vi "main-all-channels.vi"() -> ()   [LabVIEW 2024]
uses:
  controls/thermocouple-input-cluster.ctl
  controls/analog-input-cluster.ctl
  controls/analog-output-cluster.ctl
  controls/digitial-input-cluster.ctl
  controls/digital-output-cluster.ctl
  controls/adam-module-select-tab.ctl
  controls/adam-5000-serial-settings.ctl
  controls/adam-5000-cmd-response.ctl
  controls/state-enum.ctl
  controls/adam-5000-all-chassis-data.ctl
  controls/adam-5000-all-module-datas.ctl
  controls/adam-5000-chassis-cmd-ack.ctl
  controls/adam-5000-chassis-module-types.ctl
  controls/adam-5000-DO-user-input.ctl
  controls/adam-5000-AO-user-input.ctl
  <vilib>/Instr/_visa.llb/VISA Configure Serial Port (Instr).vi
  <vilib>/Instr/_visa.llb/VISA Flush IO Buffer Mask.ctl
  controls/adam-5000-module-cmd-ack.ctl
panel:
  out "cmd-response:7":T1
  out "status-indicator:7":cluster{"Sampling":bool, "Ack":bool}
  in  "Slot 7: Module Type":T2(ring)=enum."empty"
  out "slot: 7":T3
  in  "7:Digital Outputs":T4
  out "7:Digital Inputs":T5
  in  "7:Analog Outputs":T6
  out "7:Analog Inputs":T7
  out "7:Thermocouple Inputs (degC)":T8
  out "cmd-response:6":T1
  out "status-indicator:6":cluster{"Sampling":bool, "Ack":bool}
  in  "Slot 6: Module Type":T2(ring)=enum."empty"
  out "slot: 6":T3
  in  "6:Digital Outputs":T4
  out "6:Digital Inputs":T5
  in  "6:Analog Outputs":T6
  out "6:Analog Inputs":T7
  out "6:Thermocouple Inputs (degC)":T8
  out "cmd-response:5":T1
  out "status-indicator:5":cluster{"Sampling":bool, "Ack":bool}
  in  "Slot 5: Module Type":T2(ring)=enum."Analog Output"
  out "slot: 5":T3
  in  "5:Digital Outputs":T4
  out "5:Digital Inputs":T5
  in  "5:Analog Outputs":T6
  out "5:Analog Inputs":T7
  out "5:Thermocouple Inputs (degC)":T8
  out "cmd-response:4":T1
  out "status-indicator:4":cluster{"Sampling":bool, "Ack":bool}
  in  "Slot 4: Module Type":T2(ring)=enum."Power Relay"
  out "slot: 4":T3
  in  "4:Digital Outputs":T4
  out "4:Digital Inputs":T5
  in  "4:Analog Outputs":T6
  out "4:Analog Inputs":T7
  out "4:Thermocouple Inputs (degC)":T8
  out "cmd-response:3":T1
  out "status-indicator:3":cluster{"Sampling":bool, "Ack":bool}
  in  "Slot 3: Module Type":T2(ring)=enum."Thermocouple"
  out "slot: 3":T3
  in  "3:Digital Outputs":T4
  out "3:Digital Inputs":T5
  in  "3:Analog Outputs":T6
  out "3:Analog Inputs":T7
  out "3:Thermocouple Inputs (degC)":T8
  out "cmd-response:2":T1
  out "status-indicator:2":cluster{"Sampling":bool, "Ack":bool}
  in  "Slot 2: Module Type":T2(ring)=enum."Analog Input"
  out "slot: 2":T3
  in  "2:Digital Outputs":T4
  out "2:Digital Inputs":T5
  in  "2:Analog Outputs":T6
  out "2:Analog Inputs":T7
  out "2:Thermocouple Inputs (degC)":T8
  out "cmd-response:1":T1
  out "status-indicator:1":cluster{"Sampling":bool, "Ack":bool}
  in  "Slot 1: Module Type":T2(ring)=enum."Thermocouple"
  out "slot: 1":T3
  in  "1:Digital Outputs":T4
  out "1:Digital Inputs":T5
  in  "1:Analog Outputs":T6
  out "1:Analog Inputs":T7
  out "1:Thermocouple Inputs (degC)":T8
  out "cmd-response:0":T1
  out "status-indicator:0":cluster{"Sampling":bool, "Ack":bool}
  in  "Slot 0: Module Type":T2(ring)=enum."Analog Input"
  out "slot: 0":T3
  in  "0:Digital Outputs":T4
  out "0:Digital Inputs":T5
  in  "0:Analog Outputs:":T6
  out "0:Analog Inputs":T7
  out "0:Thermocouple Inputs (degC)":T8
  out "Current Slot":i32
  in  "Chassis Settings":T9={"VISA resource name"="COM8", "baud rate (19200)"=19200, "Chassis ID"=1}
  in  "Debug Mode":bool
  out "Loop Time (mS)":u32
  out "Loop Counter":i32
  out "Write Success":bool
  out "error IO":errorcluster
  out "error":errorcluster
  in  "exit":bool
  # "ADAM 5000 Controller"
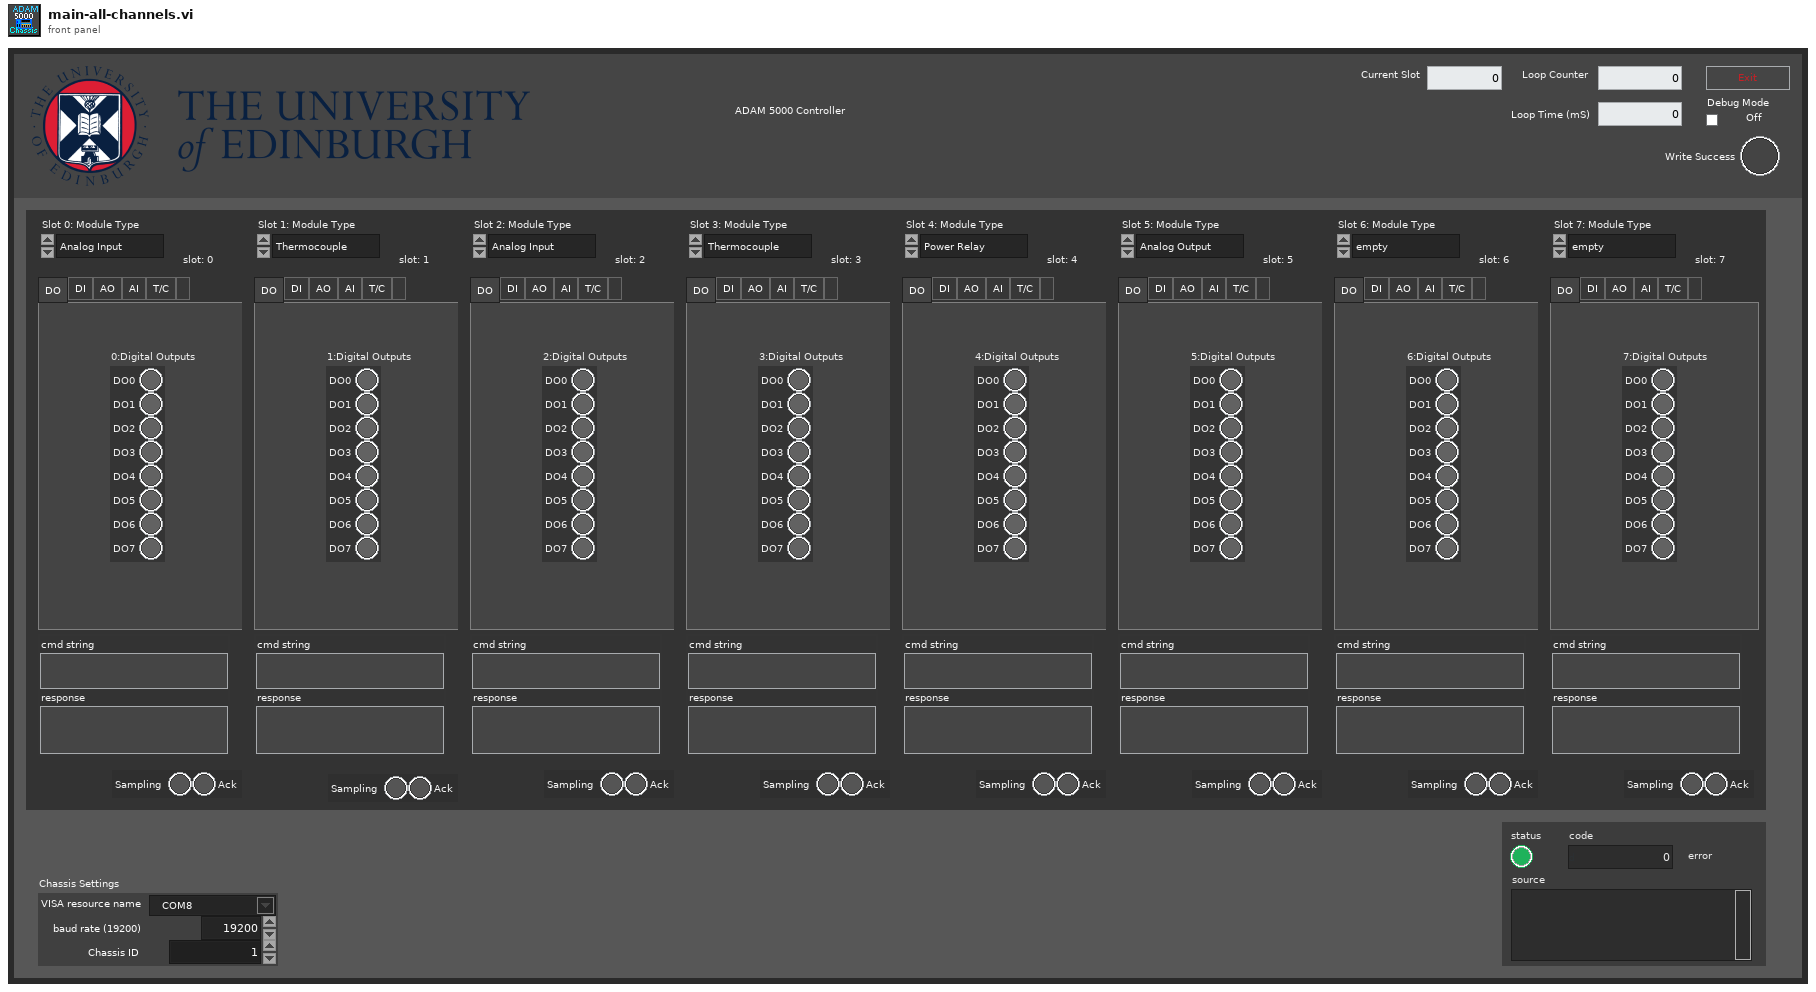
[diagram p1: front panel]
types:
  T1 = typedef "adam-5000-cmd-response.ctl" = cluster{"cmd string":string, "response":string}
  T2 = enum16{"Digital Output", "Digital Input", "Analog Output", "Analog Input", "Thermocouple", "Power Relay", "empty"}
  T3 = typedef "adam-module-select-tab.ctl" = enum32{"DO", "DI", "AO", "AI", "T/C", ""}
  T4 = typedef "digital-output-cluster.ctl" = cluster{"DO0":bool, "DO1":bool, "DO2":bool, "DO3":bool, "DO4":bool, "DO5":bool, "DO6":bool, "DO7":bool}
  T5 = typedef "digitial-input-cluster.ctl" = cluster{"DI0":bool, "DI1":bool, "DI2":bool, "DI3":bool, "DI4":bool, "DI5":bool, "DI6":bool, "DI7":bool}
  T6 = typedef "analog-output-cluster.ctl" = cluster{"AO0":dbl, "AO1":dbl, "AO2":dbl, "AO3":dbl}
  T7 = typedef "analog-input-cluster.ctl" = cluster{"AI0":dbl, "AI1":dbl, "AI2":dbl, "AI3":dbl, "AI4":dbl, "AI5":dbl, "AI6":dbl, "AI7":dbl}
  T8 = typedef "thermocouple-input-cluster.ctl" = cluster{"TC0":dbl, "TC1":dbl, "TC2":dbl, "TC3":dbl, "TC4":dbl, "TC5":dbl, "TC6":dbl}
  T9 = typedef "adam-5000-serial-settings.ctl" = cluster{"VISA resource name":refnum<visa-resource-name>, "baud rate (19200)":u32, "Chassis ID":u8}
  T10 = typedef "adam-5000-chassis-cmd-ack.ctl" = cluster{"cmd-response:0":T1, "cmd-response:1":T1, "cmd-response:2":T1, "cmd-response:3":T1, "cmd-response:4":T1, "cmd-response:5":T1, "cmd-response:6":T1, "cmd-response:7":T1}
  T11 = typedef "adam-5000-all-chassis-data.ctl" = cluster{"slot:0":T12, "slot:1":T12, "slot:2":T12, "slot:3":T12, "slot:4":T12, "slot:5":T12, "slot:6":T12, "slot:7":T12}
  T12 = typedef "adam-5000-all-module-datas.ctl" = cluster{"Digital Outputs":T4, "Digital Inputs":T5, "Analog Outputs":T6, "Analog Inputs":T7, "Thermocouple Inputs (degC)":T8}
  T13 = typedef "state-enum.ctl" = enum16{"init", "manual", "start", "run", "hold", "stop", ""}
  T14 = typedef "adam-5000-AO-user-input.ctl" = cluster{"0:Analog Outputs:":T6, "1:Analog Outputs":T6, "2:Analog Outputs":T6, "3:Analog Outputs":T6, "4:Analog Outputs":T6, "5:Analog Outputs":T6, "6:Analog Outputs":T6, "7:Analog Outputs":T6}
  T15 = typedef "adam-5000-DO-user-input.ctl" = cluster{"0:Digital Outputs":T4, "1:Digital Outputs":T4, "2:Digital Outputs":T4, "3:Digital Outputs":T4, "4:Digital Outputs":T4, "5:Digital Outputs":T4, "6:Digital Outputs":T4, "7:Digital Outputs":T4}
  T16 = typedef "adam-5000-chassis-module-types.ctl" = cluster{"Slot 0: Module Type":enum16{"Digital Output", "Digital Input", "Analog Output", "Analog Input", "Thermocouple", "Power Relay", "empty"}, "Slot 1: Module Type":enum16{"Digital Output", "Digital Input", "Analog Output", "Analog Input", "Thermocouple", "Power Relay", "empty"}, "Slot 2: Module Type":enum16{"Digital Output", "Digital Input", "Analog Output", "Analog Input", "Thermocouple", "Power Relay", "empty"}, "Slot 3: Module Type":enum16{"Digital Output", "Digital Input", "Analog Output", "Analog Input", "Thermocouple", "Power Relay", "empty"}, "Slot 4: Module Type":enum16{"Digital Output", "Digital Input", "Analog Output", "Analog Input", "Thermocouple", "Power Relay", "empty"}, "Slot 5: Module Type":enum16{"Digital Output", "Digital Input", "Analog Output", "Analog Input", "Thermocouple", "Power Relay", "empty"}, "Slot 6: Module Type":enum16{"Digital Output", "Digital Input", "Analog Output", "Analog Input", "Thermocouple", "Power Relay", "empty"}, "Slot 7: Module Type":enum16{"Digital Output", "Digital Input", "Analog Output", "Analog Input", "Thermocouple", "Power Relay", "empty"}}
  T17 = cluster{"status-indicator:0":refnum<vi>, "status-indicator:1":refnum<vi>, "status-indicator:2":refnum<vi>, "status-indicator:3":refnum<vi>, "status-indicator:4":refnum<vi>, "status-indicator:5":refnum<vi>, "status-indicator:6":refnum<vi>, "status-indicator:7":refnum<vi>}
  T18 = enum16{"Digital Output", "Digital Input", "Analog Output", "Analog Input", "Thermocouple", "Power Relay", "empty"}[]
  T19 = cluster{"[0]":T3, "[1]":T3, "[2]":T3, "[3]":T3, "[4]":T3, "[5]":T3, "[6]":T3, "[7]":T3, "[8]":T3}
  T20 = cluster{"[0]":T12, "[1]":T12, "[2]":T12, "[3]":T12, "[4]":T12, "[5]":T12, "[6]":T12, "[7]":T12, "[8]":T12}
  T21 = cluster{"[0]":T1, "[1]":T1, "[2]":T1, "[3]":T1, "[4]":T1, "[5]":T1, "[6]":T1, "[7]":T1, "[8]":T1}
  T22 = typedef "adam-5000-module-cmd-ack.ctl" = cluster{"cmd out":string, "acknowledge char":string}
  T23 = cluster{"[0]":T22, "[1]":T22, "[2]":T22, "[3]":T22, "[4]":T22, "[5]":T22, "[6]":T22, "[7]":T22, "[8]":T22}
  T24 = typedef "VISA Flush IO Buffer Mask.ctl" = u16
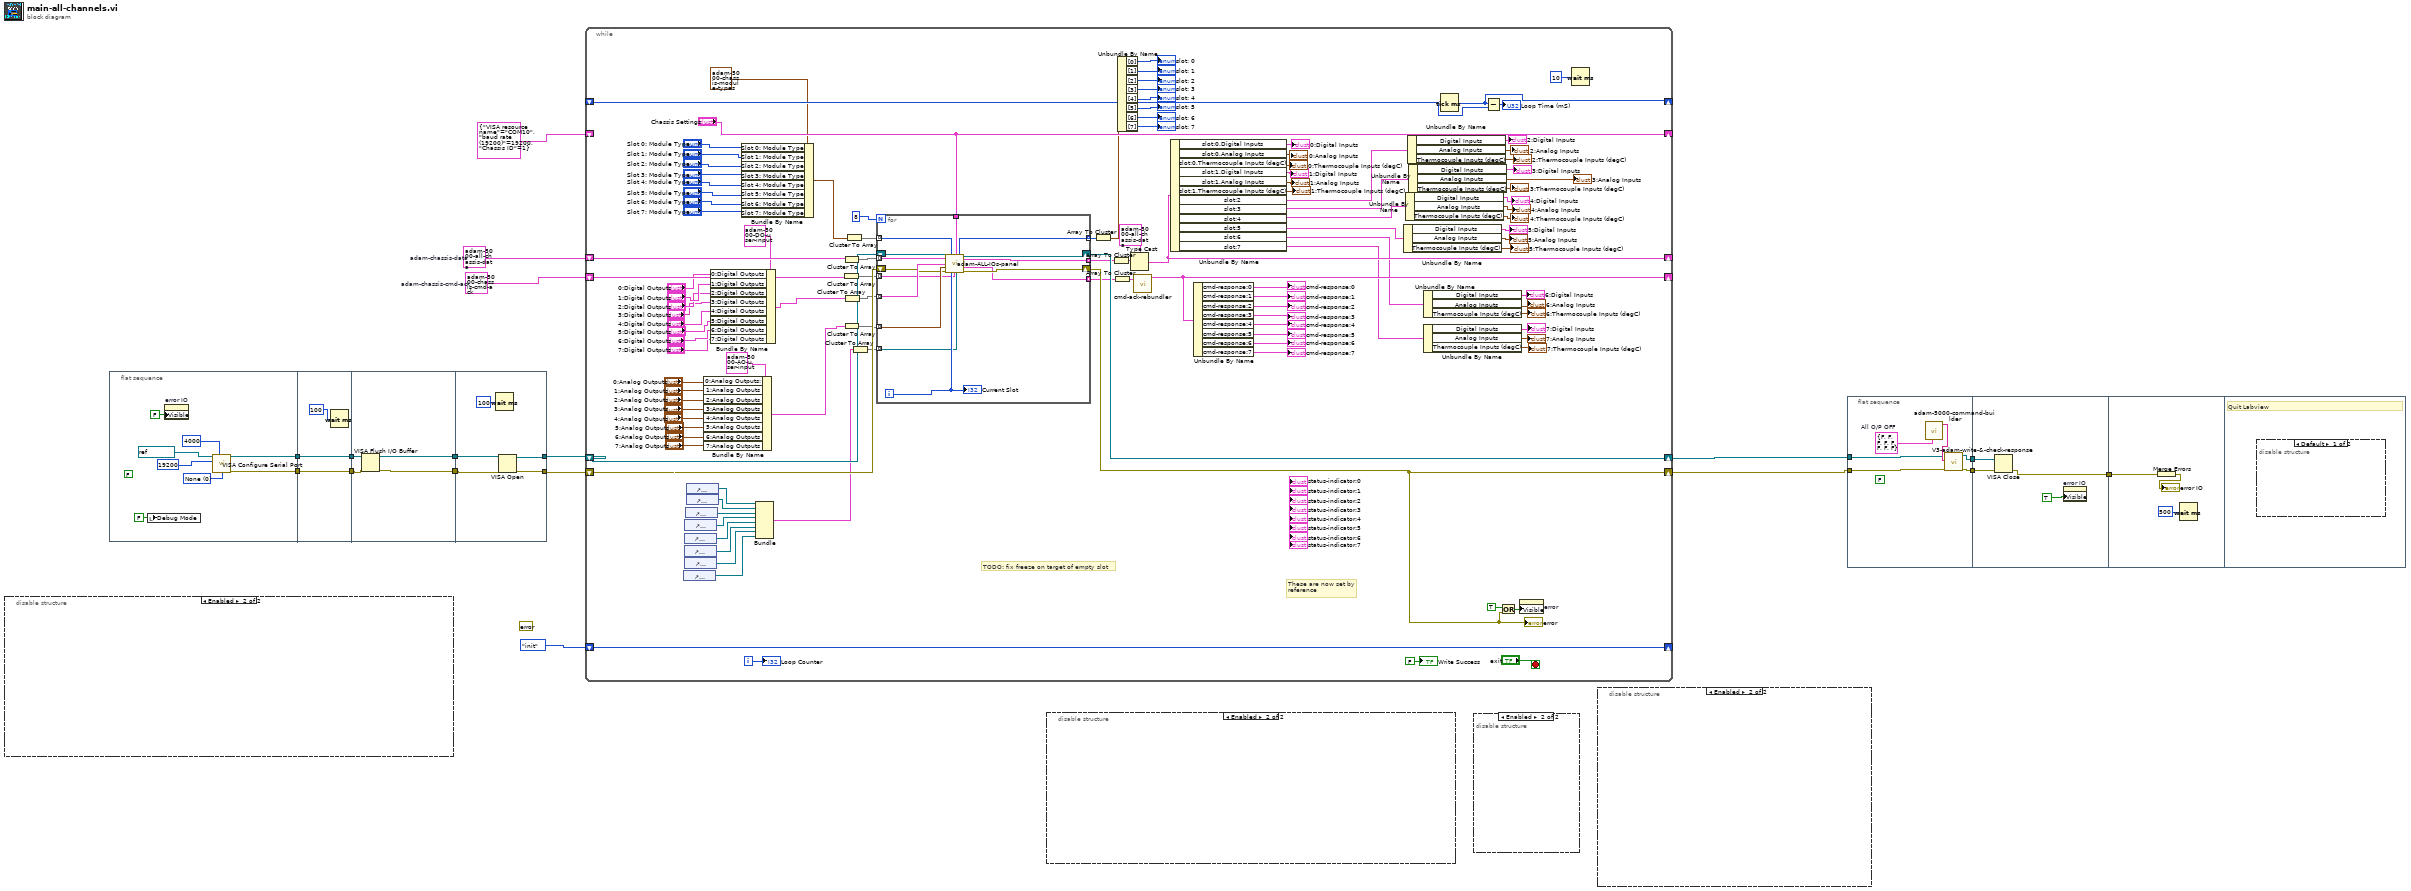
[diagram p0: block diagram]
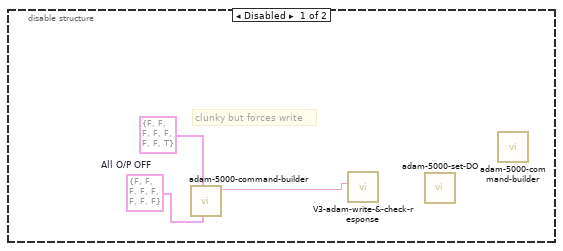
[diagram p2: hidden frame]
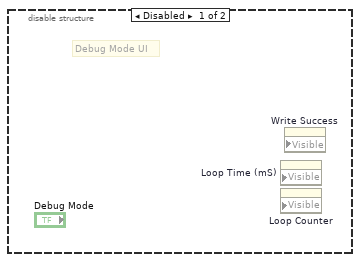
[diagram p3: hidden frame]
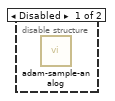
[diagram p4: hidden frame]
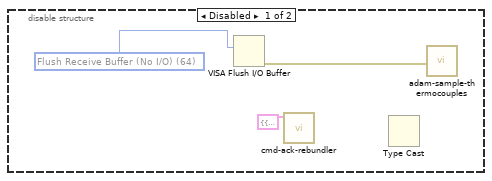
[diagram p5: hidden frame]
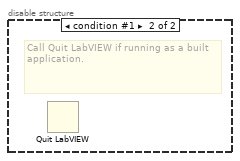
[diagram p6: hidden frame]
diagram:
  w1 = T10 {"cmd-response:0"={"cmd string"="", "response"=""}, "cmd-response:1"={"cmd string"="", "response"=""}, "cmd-response:2"={"cmd string"="", "response"=""}, "cmd-response:3"={"cmd string"="", "response"=""}, "cmd-response:4"={"cmd string"="", "response"=""}, "cmd-response:5"={"cmd string"="", "response"=""}, "cmd-response:6"={"cmd string"="", "response"=""}, "cmd-response:7"={"cmd string"="", "response"=""}}  # adam-chassis-cmd-ack
  w2 = T11 {"slot:0"={"Digital Outputs"={"DO0"=FALSE, "DO1"=FALSE, "DO2"=FALSE, "DO3"=FALSE, "DO4"=FALSE, "DO5"=FALSE, "DO6"=FALSE, "DO7"=FALSE}, "Digital Inputs"={"DI0"=FALSE, "DI1"=FALSE, "DI2"=FALSE, "DI3"=FALSE, "DI4"=FALSE, "DI5"=FALSE, "DI6"=FALSE, "DI7"=FALSE}, "Analog Outputs"={"AO0"=0.0, "AO1"=0.0, "AO2"=0.0, "AO3"=0.0}, "Analog Inputs"={"AI0"=0.0, "AI1"=0.0, "AI2"=0.0, "AI3"=0.0, "AI4"=0.0, "AI5"=0.0, "AI6"=0.0, "AI7"=0.0}, "Thermocouple Inputs (degC)"={"TC0"=0.0, "TC1"=0.0, "TC2"=0.0, "TC3"=0.0, "TC4"=0.0, "TC5"=0.0, "TC6"=0.0}}, "slot:1"={"Digital Outputs"={"DO0"=FALSE, "DO1"=FALSE, "DO2"=FALSE, "DO3"=FALSE, "DO4"=FALSE, "DO5"=FALSE, "DO6"=FALSE, "DO7"=FALSE}, "Digital Inputs"={"DI0"=FALSE, "DI1"=FALSE, "DI2"=FALSE, "DI3"=FALSE, "DI4"=FALSE, "DI5"=FALSE, "DI6"=FALSE, "DI7"=FALSE}, "Analog Outputs"={"AO0"=0.0, "AO1"=0.0, "AO2"=0.0, "AO3"=0.0}, "Analog Inputs"={"AI0"=0.0, "AI1"=0.0, "AI2"=0.0, "AI3"=0.0, "AI4"=0.0, "AI5"=0.0, "AI6"=0.0, "AI7"=0.0}, "Thermocouple Inputs (degC)"={"TC0"=0.0, "TC1"=0.0, "TC2"=0.0, "TC3"=0.0, "TC4"=0.0, "TC5"=0.0, "TC6"=0.0}}, "slot:2"={"Digital Outputs"={"DO0"=FALSE, "DO1"=FALSE, "DO2"=FALSE, "DO3"=FALSE, "DO4"=FALSE, "DO5"=FALSE, "DO6"=FALSE, "DO7"=FALSE}, "Digital Inputs"={"DI0"=FALSE, "DI1"=FALSE, "DI2"=FALSE, "DI3"=FALSE, "DI4"=FALSE, "DI5"=FALSE, "DI6"=FALSE, "DI7"=FALSE}, "Analog Outputs"={"AO0"=0.0, "AO1"=0.0, "AO2"=0.0, "AO3"=0.0}, "Analog Inputs"={"AI0"=0.0, "AI1"=0.0, "AI2"=0.0, "AI3"=0.0, "AI4"=0.0, "AI5"=0.0, "AI6"=0.0, "AI7"=0.0}, "Thermocouple Inputs (degC)"={"TC0"=0.0, "TC1"=0.0, "TC2"=0.0, "TC3"=0.0, "TC4"=0.0, "TC5"=0.0, "TC6"=0.0}}, "slot:3"={"Digital Outputs"={"DO0"=FALSE, "DO1"=FALSE, "DO2"=FALSE, "DO3"=FALSE, "DO4"=FALSE, "DO5"=FALSE, "DO6"=FALSE, "DO7"=FALSE}, "Digital Inputs"={"DI0"=FALSE, "DI1"=FALSE, "DI2"=FALSE, "DI3"=FALSE, "DI4"=FALSE, "DI5"=FALSE, "DI6"=FALSE, "DI7"=FALSE}, "Analog Outputs"={"AO0"=0.0, "AO1"=0.0, "AO2"=0.0, "AO3"=0.0}, "Analog Inputs"={"AI0"=0.0, "AI1"=0.0, "AI2"=0.0, "AI3"=0.0, "AI4"=0.0, "AI5"=0.0, "AI6"=0.0, "AI7"=0.0}, "Thermocouple Inputs (degC)"={"TC0"=0.0, "TC1"=0.0, "TC2"=0.0, "TC3"=0.0, "TC4"=0.0, "TC5"=0.0, "TC6"=0.0}}, "slot:4"={"Digital Outputs"={"DO0"=FALSE, "DO1"=FALSE, "DO2"=FALSE, "DO3"=FALSE, "DO4"=FALSE, "DO5"=FALSE, "DO6"=FALSE, "DO7"=FALSE}, "Digital Inputs"={"DI0"=FALSE, "DI1"=FALSE, "DI2"=FALSE, "DI3"=FALSE, "DI4"=FALSE, "DI5"=FALSE, "DI6"=FALSE, "DI7"=FALSE}, "Analog Outputs"={"AO0"=0.0, "AO1"=0.0, "AO2"=0.0, "AO3"=0.0}, "Analog Inputs"={"AI0"=0.0, "AI1"=0.0, "AI2"=0.0, "AI3"=0.0, "AI4"=0.0, "AI5"=0.0, "AI6"=0.0, "AI7"=0.0}, "Thermocouple Inputs (degC)"={"TC0"=0.0, "TC1"=0.0, "TC2"=0.0, "TC3"=0.0, "TC4"=0.0, "TC5"=0.0, "TC6"=0.0}}, "slot:5"={"Digital Outputs"={"DO0"=FALSE, "DO1"=FALSE, "DO2"=FALSE, "DO3"=FALSE, "DO4"=FALSE, "DO5"=FALSE, "DO6"=FALSE, "DO7"=FALSE}, "Digital Inputs"={"DI0"=FALSE, "DI1"=FALSE, "DI2"=FALSE, "DI3"=FALSE, "DI4"=FALSE, "DI5"=FALSE, "DI6"=FALSE, "DI7"=FALSE}, "Analog Outputs"={"AO0"=0.0, "AO1"=0.0, "AO2"=0.0, "AO3"=0.0}, "Analog Inputs"={"AI0"=0.0, "AI1"=0.0, "AI2"=0.0, "AI3"=0.0, "AI4"=0.0, "AI5"=0.0, "AI6"=0.0, "AI7"=0.0}, "Thermocouple Inputs (degC)"={"TC0"=0.0, "TC1"=0.0, "TC2"=0.0, "TC3"=0.0, "TC4"=0.0, "TC5"=0.0, "TC6"=0.0}}, "slot:6"={"Digital Outputs"={"DO0"=FALSE, "DO1"=FALSE, "DO2"=FALSE, "DO3"=FALSE, "DO4"=FALSE, "DO5"=FALSE, "DO6"=FALSE, "DO7"=FALSE}, "Digital Inputs"={"DI0"=FALSE, "DI1"=FALSE, "DI2"=FALSE, "DI3"=FALSE, "DI4"=FALSE, "DI5"=FALSE, "DI6"=FALSE, "DI7"=FALSE}, "Analog Outputs"={"AO0"=0.0, "AO1"=0.0, "AO2"=0.0, "AO3"=0.0}, "Analog Inputs"={"AI0"=0.0, "AI1"=0.0, "AI2"=0.0, "AI3"=0.0, "AI4"=0.0, "AI5"=0.0, "AI6"=0.0, "AI7"=0.0}, "Thermocouple Inputs (degC)"={"TC0"=0.0, "TC1"=0.0, "TC2"=0.0, "TC3"=0.0, "TC4"=0.0, "TC5"=0.0, "TC6"=0.0}}, "slot:7"={"Digital Outputs"={"DO0"=FALSE, "DO1"=FALSE, "DO2"=FALSE, "DO3"=FALSE, "DO4"=FALSE, "DO5"=FALSE, "DO6"=FALSE, "DO7"=FALSE}, "Digital Inputs"={"DI0"=FALSE, "DI1"=FALSE, "DI2"=FALSE, "DI3"=FALSE, "DI4"=FALSE, "DI5"=FALSE, "DI6"=FALSE, "DI7"=FALSE}, "Analog Outputs"={"AO0"=0.0, "AO1"=0.0, "AO2"=0.0, "AO3"=0.0}, "Analog Inputs"={"AI0"=0.0, "AI1"=0.0, "AI2"=0.0, "AI3"=0.0, "AI4"=0.0, "AI5"=0.0, "AI6"=0.0, "AI7"=0.0}, "Thermocouple Inputs (degC)"={"TC0"=0.0, "TC1"=0.0, "TC2"=0.0, "TC3"=0.0, "TC4"=0.0, "TC5"=0.0, "TC6"=0.0}}}  # adam-chassis-data
  (unwired) errorcluster {"status"=FALSE, "code"=0, "source"=""} ("error")
  n1 = disable-structure shown="Enabled" {
    frame Disabled {
      w20 = T4 {"DO0"=FALSE, "DO1"=FALSE, "DO2"=FALSE, "DO3"=FALSE, "DO4"=FALSE, "DO5"=FALSE, "DO6"=FALSE, "DO7"=FALSE}  # All O/P OFF
      # "clunky but forces write"
      n2 = call "adam-5000-command-builder.vi"("Output Control"=w20, "Current Output State"=T4 {"DO0"=FALSE, "DO1"=FALSE, "DO2"=FALSE, "DO3"=FALSE, "DO4"=FALSE, "DO5"=FALSE, "DO6"=FALSE, "DO7"=TRUE}) -> ("Command Out"=w19:string)  [unwired: 7 in, 2 out]
      n3 = call "V3-adam-write-&-check-response.vi"("write buffer"=w19) -> ("VISA resource name"=w18:refnum<visa-resource-name>)  [unwired: 5 in, 5 out]
      n4 = call "adam-5000-set-DO.vi"() -> ()  [unwired: 6 in, 6 out]
      n5 = call "adam-5000-command-builder.vi"() -> ()  [unwired: 9 in, 3 out]
    }
    frame Enabled {
    }
  }
  n6 = flat-sequence {
    tunnel: [w28] -> w11
    tunnel: [w27] -> w10
    tunnel: w11 -> [w32]
    tunnel: [w32] -> w9
    tunnel: w10 -> [w31]
    tunnel: [w31] -> w8
    tunnel: w9 -> [w36]
    tunnel: [w34] -> w7
    tunnel: w8 -> [w35]
    tunnel: [w33] -> w6
    tunnel: w7 -> [w40]
    tunnel: w6 -> [w39]
    tunnel: [w38] -> w5
    tunnel: [w37] -> w4
    frame #0 {
      w25 = u16 0 items=["None", "XON/XOFF", "RTS/CTS", "XON/XOFF & RTS/CTS", "DTR/DSR", "XON/XOFF & DTR/DSR"] ("flow control (0:none)")
      (unwired) FALSE ("V1")
      n7 = local write "Debug Mode"(FALSE ("Debug Mode")) -> ()
      n8 = property on="error IO" class="Clust (strict)"("Visible"=FALSE) -> ()  [unwired: 2 in, 2 out]
      n9 = call-poly "VISA Configure Serial Port"("VISA resource name"=refnum<visa-resource-name> "COM8", "timeout (10sec)"=u32 4000, "baud rate (9600)"=u32 19200, "flow control (0:none)"=w25) -> ("VISA resource name out"=w28:refnum<visa-resource-name>, "error out"=w27:errorcluster)  [unwired: 10 in]
    }
    frame #1 {
      n10 = Wait (ms)(milliseconds to wait=u32 100) -> ()  [unwired: 1 out]
    }
    frame #2 {
      n11 = VISA Flush I/O Buffer(VISA resource name=w36, error in (no error)=w35) -> (VISA resource name out=w34:refnum<visa-resource-name>, error out=w33:errorcluster)  [unwired: 1 in]
    }
    frame #3 {
      n12 = Wait (ms)(milliseconds to wait=u32 100) -> ()  [unwired: 1 out]
      n13 = VISA Open(error in (no error)=w39, VISA resource name=w40) -> (VISA resource name=w38:refnum<visa-resource-name>, error out=w37:errorcluster)  [unwired: 3 in]
    }
  }
  n14 = while {
    shift-right: [w151] -> _
    shift-left: state-enum."init" ("state-enum") -> [w151]
    shift-right: [w127] -> w16
    shift-left: w4 -> [w139]
    shift-right: [w154] -> _
    shift-left: _ -> [w156]
    shift-right: ["Chassis Settings"] -> _
    shift-left: T9 {"VISA resource name"="COM10", "baud rate (19200)"=19200, "Chassis ID"=1} ("Chassis Settings") -> [_]
    shift-right: [w138] -> w3
    shift-left: w5 -> [w140]
    shift-right: [w128] -> _
    shift-left: w2 -> [w137]
    shift-right: [w112] -> _
    shift-left: w1 -> [w135]
    i -> [w157]
    stop <- "exit" stop-if-true
    # "TODO: fix freeze on target of empty slot"
    # "These are now set by\nreference"
    n15 = control-ref of="status-indicator:7"() -> (w72:refnum<vi>)
    n16 = control-ref of="status-indicator:4"() -> (w75:refnum<vi>)
    n17 = control-ref of="status-indicator:5"() -> (w74:refnum<vi>)
    n18 = control-ref of="status-indicator:3"() -> (w76:refnum<vi>)
    n19 = control-ref of="status-indicator:6"() -> (w73:refnum<vi>)
    n20 = control-ref of="status-indicator:2"() -> (w106:refnum<vi>)
    n21 = control-ref of="status-indicator:0"() -> (w124:refnum<vi>)
    n22 = control-ref of="status-indicator:1"() -> (w123:refnum<vi>)
    n23 = Bundle By Name(cluster=T14 {"0:Analog Outputs:"={"AO0"=0.0, "AO1"=0.0, "AO2"=0.0, "AO3"=0.0}, "1:Analog Outputs"={"AO0"=0.0, "AO1"=0.0, "AO2"=0.0, "AO3"=0.0}, "2:Analog Outputs"={"AO0"=0.0, "AO1"=0.0, "AO2"=0.0, "AO3"=0.0}, "3:Analog Outputs"={"AO0"=0.0, "AO1"=0.0, "AO2"=0.0, "AO3"=0.0}, "4:Analog Outputs"={"AO0"=0.0, "AO1"=0.0, "AO2"=0.0, "AO3"=0.0}, "5:Analog Outputs"={"AO0"=0.0, "AO1"=0.0, "AO2"=0.0, "AO3"=0.0}, "6:Analog Outputs"={"AO0"=0.0, "AO1"=0.0, "AO2"=0.0, "AO3"=0.0}, "7:Analog Outputs"={"AO0"=0.0, "AO1"=0.0, "AO2"=0.0, "AO3"=0.0}}, "0:Analog Outputs:"="0:Analog Outputs:", "1:Analog Outputs"="1:Analog Outputs", "2:Analog Outputs"="2:Analog Outputs", "3:Analog Outputs"="3:Analog Outputs", "4:Analog Outputs"="4:Analog Outputs", "5:Analog Outputs"="5:Analog Outputs", "6:Analog Outputs"="6:Analog Outputs", "7:Analog Outputs"="7:Analog Outputs") -> (w50:T14)
    n24 = Bundle By Name(cluster=T15 {"0:Digital Outputs"={"DO0"=FALSE, "DO1"=FALSE, "DO2"=FALSE, "DO3"=FALSE, "DO4"=FALSE, "DO5"=FALSE, "DO6"=FALSE, "DO7"=FALSE}, "1:Digital Outputs"={"DO0"=FALSE, "DO1"=FALSE, "DO2"=FALSE, "DO3"=FALSE, "DO4"=FALSE, "DO5"=FALSE, "DO6"=FALSE, "DO7"=FALSE}, "2:Digital Outputs"={"DO0"=FALSE, "DO1"=FALSE, "DO2"=FALSE, "DO3"=FALSE, "DO4"=FALSE, "DO5"=FALSE, "DO6"=FALSE, "DO7"=FALSE}, "3:Digital Outputs"={"DO0"=FALSE, "DO1"=FALSE, "DO2"=FALSE, "DO3"=FALSE, "DO4"=FALSE, "DO5"=FALSE, "DO6"=FALSE, "DO7"=FALSE}, "4:Digital Outputs"={"DO0"=FALSE, "DO1"=FALSE, "DO2"=FALSE, "DO3"=FALSE, "DO4"=FALSE, "DO5"=FALSE, "DO6"=FALSE, "DO7"=FALSE}, "5:Digital Outputs"={"DO0"=FALSE, "DO1"=FALSE, "DO2"=FALSE, "DO3"=FALSE, "DO4"=FALSE, "DO5"=FALSE, "DO6"=FALSE, "DO7"=FALSE}, "6:Digital Outputs"={"DO0"=FALSE, "DO1"=FALSE, "DO2"=FALSE, "DO3"=FALSE, "DO4"=FALSE, "DO5"=FALSE, "DO6"=FALSE, "DO7"=FALSE}, "7:Digital Outputs"={"DO0"=FALSE, "DO1"=FALSE, "DO2"=FALSE, "DO3"=FALSE, "DO4"=FALSE, "DO5"=FALSE, "DO6"=FALSE, "DO7"=FALSE}}, "0:Digital Outputs"="0:Digital Outputs", "1:Digital Outputs"="1:Digital Outputs", "2:Digital Outputs"="2:Digital Outputs", "3:Digital Outputs"="3:Digital Outputs", "4:Digital Outputs"="4:Digital Outputs", "5:Digital Outputs"="5:Digital Outputs", "6:Digital Outputs"="6:Digital Outputs", "7:Digital Outputs"="7:Digital Outputs") -> (w60:T15)
    n25 = Bundle By Name(cluster=T16 {"Slot 0: Module Type"=enum."Digital Output", "Slot 1: Module Type"=enum."Digital Output", "Slot 2: Module Type"=enum."Digital Output", "Slot 3: Module Type"=enum."Digital Output", "Slot 4: Module Type"=enum."Digital Output", "Slot 5: Module Type"=enum."Digital Output", "Slot 6: Module Type"=enum."Digital Output", "Slot 7: Module Type"=enum."Digital Output"}, "Slot 0: Module Type"="Slot 0: Module Type", "Slot 1: Module Type"="Slot 1: Module Type", "Slot 2: Module Type"="Slot 2: Module Type", "Slot 3: Module Type"="Slot 3: Module Type", "Slot 4: Module Type"="Slot 4: Module Type", "Slot 5: Module Type"="Slot 5: Module Type", "Slot 6: Module Type"="Slot 6: Module Type", "Slot 7: Module Type"="Slot 7: Module Type") -> (w62:T16)
    n26 = Bundle("status-indicator:0"=w124, "status-indicator:1"=w123, "status-indicator:2"=w106, "status-indicator:3"=w76, "status-indicator:4"=w75, "status-indicator:5"=w74, "status-indicator:6"=w73, "status-indicator:7"=w72) -> (w122:T17)  [unwired: 1 in]
    n27 = Cluster To Array(cluster=w135) -> (array=w134:T1[])
    n28 = Cluster To Array(cluster=w137) -> (array=w136:T12[])
    n29 = Cluster To Array(cluster=w50) -> (array=w132:T6[])
    n30 = Cluster To Array(cluster=w60) -> (array=w133:T4[])
    n31 = Cluster To Array(cluster=w62) -> (array=w126:T18)
    n32 = Cluster To Array(cluster=w122) -> (array=w121:refnum<vi>[])
    n33 = for {
      N: 8 -> [_]
      shift-right: [w165] -> w127
      shift-left: w139 -> [w166]
      shift-right: [w171] -> w138
      shift-left: w140 -> [w170]
      tunnel: w136 -> [w169] mode=indexing
      tunnel: w134 -> [w161] mode=indexing
      tunnel: w133 -> [w168] mode=indexing
      tunnel: w132 -> [w167] mode=indexing
      tunnel: "Chassis Settings" -> [w173]
      tunnel: w126 -> [w174] mode=indexing
      tunnel: w121 -> [w160] mode=indexing
      tunnel: [w172] -> w120 mode=indexing
      tunnel: [w164] -> w119 mode=indexing
      tunnel: [w163] -> w118 mode=indexing
      i -> [w162]
      n34 = call "adam-ALL-IOs-panel.vi"("VISA Refnum in"=w170, "ADAM-5000-data-current"=w169, "Digital Outputs"=w168, "Analog Outputs"=w167, "error in (no error)"=w166, "Module Type"=w174, "chassis-slot"=w162, "cmd-response in"=w161, "Chassis Settings"=w173, "reference"=w160) -> ("slot: x"=w172:T3, "VISA Refnum out"=w171:refnum<visa-resource-name>, "ADAM-5000-data-new"=w164:T12, "cmd-response out"=w163:T1, "error out"=w165:errorcluster)  [unwired: 5 in]
      "Current Slot" <- w162
    }
    "error" <- w127
    n35 = Array To Cluster(array=w120) -> (cluster=w125:T19)
    n36 = Array To Cluster(array=w119) -> (cluster=w130:T20)
    n37 = Array To Cluster(array=w118) -> (cluster=w111:T21)
    n38 = Unbundle By Name(w125) -> ("[0]"=→"slot: 0":T3, "[1]"=→"slot: 1":T3, "[2]"=→"slot: 2":T3, "[3]"=→"slot: 3":T3, "[4]"=→"slot: 4":T3, "[5]"=→"slot: 5":T3, "[6]"=→"slot: 6":T3, "[7]"=→"slot: 7":T3)
    n39 = Type Cast(type=T11 {"slot:0"={"Digital Outputs"={"DO0"=FALSE, "DO1"=FALSE, "DO2"=FALSE, "DO3"=FALSE, "DO4"=FALSE, "DO5"=FALSE, "DO6"=FALSE, "DO7"=FALSE}, "Digital Inputs"={"DI0"=FALSE, "DI1"=FALSE, "DI2"=FALSE, "DI3"=FALSE, "DI4"=FALSE, "DI5"=FALSE, "DI6"=FALSE, "DI7"=FALSE}, "Analog Outputs"={"AO0"=0.0, "AO1"=0.0, "AO2"=0.0, "AO3"=0.0}, "Analog Inputs"={"AI0"=0.0, "AI1"=0.0, "AI2"=0.0, "AI3"=0.0, "AI4"=0.0, "AI5"=0.0, "AI6"=0.0, "AI7"=0.0}, "Thermocouple Inputs (degC)"={"TC0"=0.0, "TC1"=0.0, "TC2"=0.0, "TC3"=0.0, "TC4"=0.0, "TC5"=0.0, "TC6"=0.0}}, "slot:1"={"Digital Outputs"={"DO0"=FALSE, "DO1"=FALSE, "DO2"=FALSE, "DO3"=FALSE, "DO4"=FALSE, "DO5"=FALSE, "DO6"=FALSE, "DO7"=FALSE}, "Digital Inputs"={"DI0"=FALSE, "DI1"=FALSE, "DI2"=FALSE, "DI3"=FALSE, "DI4"=FALSE, "DI5"=FALSE, "DI6"=FALSE, "DI7"=FALSE}, "Analog Outputs"={"AO0"=0.0, "AO1"=0.0, "AO2"=0.0, "AO3"=0.0}, "Analog Inputs"={"AI0"=0.0, "AI1"=0.0, "AI2"=0.0, "AI3"=0.0, "AI4"=0.0, "AI5"=0.0, "AI6"=0.0, "AI7"=0.0}, "Thermocouple Inputs (degC)"={"TC0"=0.0, "TC1"=0.0, "TC2"=0.0, "TC3"=0.0, "TC4"=0.0, "TC5"=0.0, "TC6"=0.0}}, "slot:2"={"Digital Outputs"={"DO0"=FALSE, "DO1"=FALSE, "DO2"=FALSE, "DO3"=FALSE, "DO4"=FALSE, "DO5"=FALSE, "DO6"=FALSE, "DO7"=FALSE}, "Digital Inputs"={"DI0"=FALSE, "DI1"=FALSE, "DI2"=FALSE, "DI3"=FALSE, "DI4"=FALSE, "DI5"=FALSE, "DI6"=FALSE, "DI7"=FALSE}, "Analog Outputs"={"AO0"=0.0, "AO1"=0.0, "AO2"=0.0, "AO3"=0.0}, "Analog Inputs"={"AI0"=0.0, "AI1"=0.0, "AI2"=0.0, "AI3"=0.0, "AI4"=0.0, "AI5"=0.0, "AI6"=0.0, "AI7"=0.0}, "Thermocouple Inputs (degC)"={"TC0"=0.0, "TC1"=0.0, "TC2"=0.0, "TC3"=0.0, "TC4"=0.0, "TC5"=0.0, "TC6"=0.0}}, "slot:3"={"Digital Outputs"={"DO0"=FALSE, "DO1"=FALSE, "DO2"=FALSE, "DO3"=FALSE, "DO4"=FALSE, "DO5"=FALSE, "DO6"=FALSE, "DO7"=FALSE}, "Digital Inputs"={"DI0"=FALSE, "DI1"=FALSE, "DI2"=FALSE, "DI3"=FALSE, "DI4"=FALSE, "DI5"=FALSE, "DI6"=FALSE, "DI7"=FALSE}, "Analog Outputs"={"AO0"=0.0, "AO1"=0.0, "AO2"=0.0, "AO3"=0.0}, "Analog Inputs"={"AI0"=0.0, "AI1"=0.0, "AI2"=0.0, "AI3"=0.0, "AI4"=0.0, "AI5"=0.0, "AI6"=0.0, "AI7"=0.0}, "Thermocouple Inputs (degC)"={"TC0"=0.0, "TC1"=0.0, "TC2"=0.0, "TC3"=0.0, "TC4"=0.0, "TC5"=0.0, "TC6"=0.0}}, "slot:4"={"Digital Outputs"={"DO0"=FALSE, "DO1"=FALSE, "DO2"=FALSE, "DO3"=FALSE, "DO4"=FALSE, "DO5"=FALSE, "DO6"=FALSE, "DO7"=FALSE}, "Digital Inputs"={"DI0"=FALSE, "DI1"=FALSE, "DI2"=FALSE, "DI3"=FALSE, "DI4"=FALSE, "DI5"=FALSE, "DI6"=FALSE, "DI7"=FALSE}, "Analog Outputs"={"AO0"=0.0, "AO1"=0.0, "AO2"=0.0, "AO3"=0.0}, "Analog Inputs"={"AI0"=0.0, "AI1"=0.0, "AI2"=0.0, "AI3"=0.0, "AI4"=0.0, "AI5"=0.0, "AI6"=0.0, "AI7"=0.0}, "Thermocouple Inputs (degC)"={"TC0"=0.0, "TC1"=0.0, "TC2"=0.0, "TC3"=0.0, "TC4"=0.0, "TC5"=0.0, "TC6"=0.0}}, "slot:5"={"Digital Outputs"={"DO0"=FALSE, "DO1"=FALSE, "DO2"=FALSE, "DO3"=FALSE, "DO4"=FALSE, "DO5"=FALSE, "DO6"=FALSE, "DO7"=FALSE}, "Digital Inputs"={"DI0"=FALSE, "DI1"=FALSE, "DI2"=FALSE, "DI3"=FALSE, "DI4"=FALSE, "DI5"=FALSE, "DI6"=FALSE, "DI7"=FALSE}, "Analog Outputs"={"AO0"=0.0, "AO1"=0.0, "AO2"=0.0, "AO3"=0.0}, "Analog Inputs"={"AI0"=0.0, "AI1"=0.0, "AI2"=0.0, "AI3"=0.0, "AI4"=0.0, "AI5"=0.0, "AI6"=0.0, "AI7"=0.0}, "Thermocouple Inputs (degC)"={"TC0"=0.0, "TC1"=0.0, "TC2"=0.0, "TC3"=0.0, "TC4"=0.0, "TC5"=0.0, "TC6"=0.0}}, "slot:6"={"Digital Outputs"={"DO0"=FALSE, "DO1"=FALSE, "DO2"=FALSE, "DO3"=FALSE, "DO4"=FALSE, "DO5"=FALSE, "DO6"=FALSE, "DO7"=FALSE}, "Digital Inputs"={"DI0"=FALSE, "DI1"=FALSE, "DI2"=FALSE, "DI3"=FALSE, "DI4"=FALSE, "DI5"=FALSE, "DI6"=FALSE, "DI7"=FALSE}, "Analog Outputs"={"AO0"=0.0, "AO1"=0.0, "AO2"=0.0, "AO3"=0.0}, "Analog Inputs"={"AI0"=0.0, "AI1"=0.0, "AI2"=0.0, "AI3"=0.0, "AI4"=0.0, "AI5"=0.0, "AI6"=0.0, "AI7"=0.0}, "Thermocouple Inputs (degC)"={"TC0"=0.0, "TC1"=0.0, "TC2"=0.0, "TC3"=0.0, "TC4"=0.0, "TC5"=0.0, "TC6"=0.0}}, "slot:7"={"Digital Outputs"={"DO0"=FALSE, "DO1"=FALSE, "DO2"=FALSE, "DO3"=FALSE, "DO4"=FALSE, "DO5"=FALSE, "DO6"=FALSE, "DO7"=FALSE}, "Digital Inputs"={"DI0"=FALSE, "DI1"=FALSE, "DI2"=FALSE, "DI3"=FALSE, "DI4"=FALSE, "DI5"=FALSE, "DI6"=FALSE, "DI7"=FALSE}, "Analog Outputs"={"AO0"=0.0, "AO1"=0.0, "AO2"=0.0, "AO3"=0.0}, "Analog Inputs"={"AI0"=0.0, "AI1"=0.0, "AI2"=0.0, "AI3"=0.0, "AI4"=0.0, "AI5"=0.0, "AI6"=0.0, "AI7"=0.0}, "Thermocouple Inputs (degC)"={"TC0"=0.0, "TC1"=0.0, "TC2"=0.0, "TC3"=0.0, "TC4"=0.0, "TC5"=0.0, "TC6"=0.0}}}, x=w130) -> (*(type *) &x=w128:T11)
    n40 = call "cmd-ack-rebundler.vi"("cmd-response-in"=w111) -> ("adam-chassis-cmd-response-out"=w112:T10)  [unwired: 10 in]
    n41 = Unbundle By Name(w128) -> ("slot:0.Digital Inputs"=→"0:Digital Inputs":T5, "slot:0.Analog Inputs"=→"0:Analog Inputs":T7, "slot:0.Thermocouple Inputs (degC)"=→"0:Thermocouple Inputs (degC)":T8, "slot:1.Digital Inputs"=→"1:Digital Inputs":T5, "slot:1.Analog Inputs"=→"1:Analog Inputs":T7, "slot:1.Thermocouple Inputs (degC)"=→"1:Thermocouple Inputs (degC)":T8, "slot:2"=w116:T12, "slot:3"=w107:T12, "slot:4"=w101:T12, "slot:5"=w88:T12, "slot:6"=w84:T12, "slot:7"=w83:T12)
    n42 = Unbundle By Name(w112) -> ("cmd-response:0"=→"cmd-response:0":T1, "cmd-response:1"=→"cmd-response:1":T1, "cmd-response:2"=→"cmd-response:2":T1, "cmd-response:3"=→"cmd-response:3":T1, "cmd-response:4"=→"cmd-response:4":T1, "cmd-response:5"=→"cmd-response:5":T1, "cmd-response:6"=→"cmd-response:6":T1, "cmd-response:7"=→"cmd-response:7":T1)
    n43 = Unbundle By Name(w88) -> ("Digital Inputs"=→"5:Digital Inputs":T5, "Analog Inputs"=→"5:Analog Inputs":T7, "Thermocouple Inputs (degC)"=→"5:Thermocouple Inputs (degC)":T8)
    n44 = Unbundle By Name(w101) -> ("Digital Inputs"=→"4:Digital Inputs":T5, "Analog Inputs"=→"4:Analog Inputs":T7, "Thermocouple Inputs (degC)"=→"4:Thermocouple Inputs (degC)":T8)
    n45 = Unbundle By Name(w116) -> ("Digital Inputs"=→"2:Digital Inputs":T5, "Analog Inputs"=→"2:Analog Inputs":T7, "Thermocouple Inputs (degC)"=→"2:Thermocouple Inputs (degC)":T8)
    n46 = Unbundle By Name(w107) -> ("Digital Inputs"=→"3:Digital Inputs":T5, "Analog Inputs"=→"3:Analog Inputs":T7, "Thermocouple Inputs (degC)"=→"3:Thermocouple Inputs (degC)":T8)
    n47 = Unbundle By Name(w84) -> ("Digital Inputs"=→"6:Digital Inputs":T5, "Analog Inputs"=→"6:Analog Inputs":T7, "Thermocouple Inputs (degC)"=→"6:Thermocouple Inputs (degC)":T8)
    n48 = Unbundle By Name(w83) -> ("Digital Inputs"=→"7:Digital Inputs":T5, "Analog Inputs"=→"7:Analog Inputs":T7, "Thermocouple Inputs (degC)"=→"7:Thermocouple Inputs (degC)":T8)
    n49 = Tick Count (ms)() -> (millisecond timer value=w154:u32)
    n50 = Subtract(x=w154, y=w156) -> (x-y=→"Loop Time (mS)":u32)
    n51 = Or(x=TRUE ("Debug Mode"), y=w127) -> (x .or. y?=w153:bool)
    n52 = property on="error" class="Clust (strict)"("Visible"=w153) -> ()  [unwired: 2 in, 2 out]
    n53 = Wait (ms)(milliseconds to wait=u32 10) -> ()  [unwired: 1 out]
    "Write Success" <- FALSE ("Write Success")
    "Loop Counter" <- w157
  }
  n54 = disable-structure shown="Enabled" {
    frame Disabled {
      w180 = T24 64 items=["Flush Receive Buffer"=16, "Write Transmit Buffer to Device"=32, "Flush Receive Buffer (No I/O)"=64, "Flush Transmit Buffer"=128] ("Mask")
      n55 = VISA Flush I/O Buffer(mask (16)=w180) -> (error out=w179:errorcluster)  [unwired: 2 in, 1 out]
      n56 = call "cmd-ack-rebundler.vi"("adam-chassis-cmd-response-in"=T23 {"[0]"={"cmd out"="", "acknowledge char"=""}, "[1]"={"cmd out"="", "acknowledge char"=""}, "[2]"={"cmd out"="", "acknowledge char"=""}, "[3]"={"cmd out"="", "acknowledge char"=""}, "[4]"={"cmd out"="", "acknowledge char"=""}, "[5]"={"cmd out"="", "acknowledge char"=""}, "[6]"={"cmd out"="", "acknowledge char"=""}, "[7]"={"cmd out"="", "acknowledge char"=""}, "[8]"={"cmd out"="", "acknowledge char"=""}} ("cmd-ack-in")) -> ()  [unwired: 10 in, 1 out]
      n57 = Type Cast() -> ()  [unwired: 2 in, 1 out]
      n58 = call "adam-sample-thermocouples.vi"("error in (no error)"=w179) -> ("status"=w177:string, "read buffer"=w176:string, "acknowledge char"=w178:string)  [unwired: 5 in, 3 out]
    }
    frame Enabled {
    }
  }
  n59 = disable-structure shown="Enabled" {
    frame Disabled {
      n60 = call "adam-sample-analog.vi"() -> ()  [unwired: 6 in, 6 out]
    }
    frame Enabled {
    }
  }
  n61 = disable-structure shown="Enabled" {
    frame Disabled {
      # "Debug Mode UI"
      n62 = property on="Loop Time (mS)" class="DigNum (strict)" props=["Visible"]() -> ()  [unwired: 3 in, 2 out]
      n63 = property on="Loop Counter" class="DigNum (strict)" props=["Visible"]() -> ()  [unwired: 3 in, 2 out]
      n64 = property on="Write Success" class="Bool (strict)" props=["Visible"]() -> ()  [unwired: 3 in, 2 out]
    }
    frame Enabled {
    }
  }
  n65 = flat-sequence {
    tunnel: w16 -> [w186]
    tunnel: [w185] -> w14
    tunnel: [w184] -> w13
    tunnel: w3 -> [w182]
    tunnel: [w188] -> w15
    tunnel: w14 -> [w189]
    tunnel: w13 -> [w190]
    tunnel: w15 -> [w192]
    frame #0 {
      (unwired) FALSE ("V1")
      w183 = T4 {"DO0"=FALSE, "DO1"=FALSE, "DO2"=FALSE, "DO3"=FALSE, "DO4"=FALSE, "DO5"=FALSE, "DO6"=FALSE, "DO7"=FALSE}  # All O/P OFF
      n66 = call "adam-5000-command-builder.vi"("Output Control"=w183) -> ("Command Out"=w187:string)  [unwired: 8 in, 2 out]
      n67 = call "V3-adam-write-&-check-response.vi"("error in (no error)"=w186, "write buffer"=w187, "VISA resource name"=w182) -> ("error out"=w184:errorcluster, "VISA resource name out"=w185:refnum<visa-resource-name>)  [unwired: 4 in, 3 out]
    }
    frame #1 {
      n68 = VISA Close(VISA resource name=w189, error in (no error)=w190) -> (error out=w188:errorcluster)
      n69 = property on="error IO" class="Clust (strict)"("Visible"=TRUE) -> ()  [unwired: 2 in, 2 out]
    }
    frame #2 {
      n70 = Merge Errors(w192) -> (→"error IO":errorcluster)
      n71 = Wait (ms)(milliseconds to wait=u32 500) -> ()  [unwired: 1 out]
    }
    frame #3 {
      # "Quit Labview"
      n72 = disable-structure "Conditional Disable Structure" shown="Default" {
        frame condition #0 (active) {
        }
        frame condition #1 {
          # "Call Quit LabVIEW if running as a built application."
          n73 = Quit LabVIEW() -> ()  [unwired: 1 in]
        }
      }
    }
  }
